vi "Exemple_Metrics_Multilabel_Confusion_Matrix.vi"() -> ()   [LabVIEW 2020]
uses:
  Objet/3 - Model selection and evaluation/3.3 - Metrics and scoring/multilabel_confusion_matrix/Multilabel_Confusion_Matrix.vi
panel:
  out "Data":T1
  out "error out":errorcluster caption="sortie d'erreur"
  in  "multilabel_confusion_matrix":T2={"sample_weight"=[], "labels"={"dtype_labels"="None", "labels"=["None"]}, "samplewise"=FALSE}
  in  "error in (no error)":errorcluster caption="entrée d'erreur (pas d'erreur)"
  in  "y_pred":string[][](array[string])=[["1", "0", "0"], ["0", "1", "1"]]
  in  "y_true":string[][](array[string])=[["1", "0", "1"], ["0", "1", "0"]]
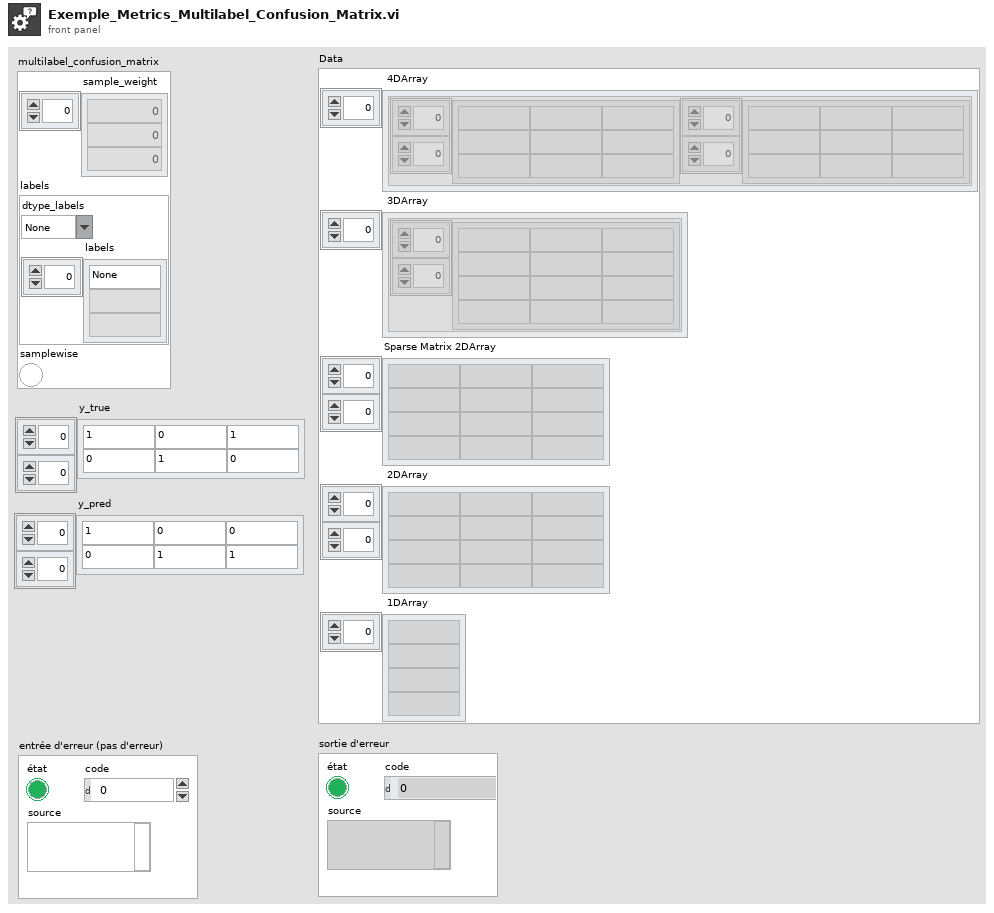
[diagram p1: front panel]
types:
  T1 = cluster{" 4DArray":cluster{"1":string[][], "2":string[][]}[], " 3DArray":cluster{"Tableau":string[][]}[], "Sparse Matrix 2DArray":string[][], " 2DArray":string[][], " 1DArray":string[]}
  T2 = cluster{"sample_weight":dbl[], "labels":cluster{"dtype_labels":string, "labels":string[]}, "samplewise":bool}
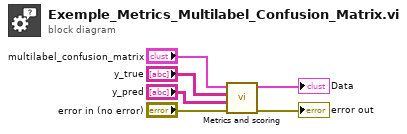
[diagram p0: block diagram]
diagram:
  n1 = call-poly "Metrics and scoring.vi"("error in (no error)"="error in (no error)", "y_pred"="y_pred", "y_true"="y_true", "multilabel_confusion_matrix"="multilabel_confusion_matrix") -> ("error out"=→"error out":errorcluster, "Data"=→"Data":T1)  [unwired: 6 in]
